vi "Sensor.vi"   [LabVIEW 2014, in "Sensors.lvlib" / "Sensor.lvclass"]
uses:
  Sensor.lvclass
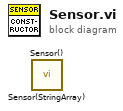
[diagram p0: block diagram]
diagram:
  n1 = call "Sensor(StringArray).vi"() -> ()  [unwired: 11 in, 1 out]
  n2 = call "Sensor().vi"() -> ()  [unwired: 11 in, 1 out]
